vi "Track Written and Read DRAM Bytes.vi"(0 "write valid":bool, 1 "reset":bool, 5 "read valid":bool, 7 "flush":bool) -> (4 "bytes written":u64, 6 "bytes read":u64, 8 "last byte flushed":bool)   [LabVIEW 2020, in "GettingStarted_Common_148X_FPGA.lvlib"]
uses:
  GettingStarted_Common_148X_FPGA.lvlib
  <instrlib>/_niInstr/Basic Elements/v1/FPGA/Private/Count Up U64.vi
  <instrlib>/_niInstr/Basic Elements/v1/FPGA/niInstr Basic Elements v1 FPGA.lvlib
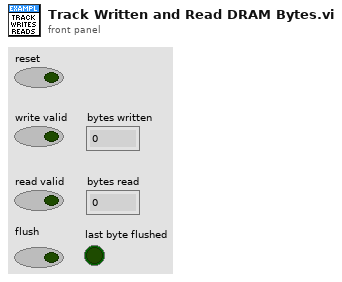
[diagram p1: front panel]
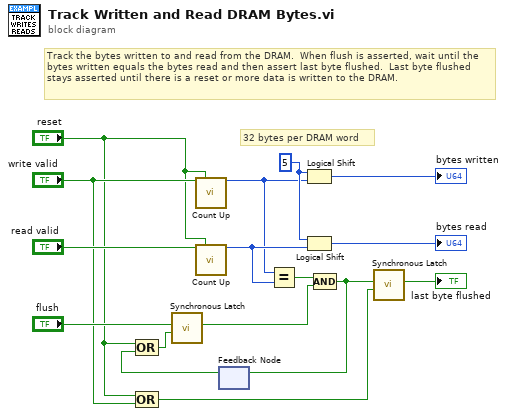
[diagram p0: block diagram]
diagram:
  w15 = i16 5 ("y")
  # "Track the bytes written to and read from the DRAM.  When flush is asserted, wait until the bytes written equals the bytes read and then assert last byte flushed.  Last byte flushed stays asserted until there is a reset or more data is written to the DRAM."
  # "32 bytes per DRAM word"
  n1 = Compound Arithmetic op=OR("reset", "write valid") -> (w7:bool)
  n2 = call-poly <instrlib>:"Count Up.vi"("increment"="write valid", "reset"="reset") -> ("count out"=w3:u64)  [unwired: 13 in]
  n3 = call-poly <instrlib>:"Count Up.vi"("increment"="read valid", "reset"="reset") -> ("count out"=w5:u64)  [unwired: 13 in]
  n4 = feedback #1() -> (w11:bool)  [unwired: 1 in]
  n5 = Compound Arithmetic op=OR("reset", w11) -> (w14:bool)
  n6 = call <instrlib>:"Synchronous Latch.vi"("clear"=w14, "set"="flush") -> ("out"=w10:bool)  [unwired: 9 in]
  n7 = Equal?(x=w3, y=w5) -> (x = y?=w12:bool)
  n8 = Logical Shift(y=w15, x=w3) -> (x << y=→"bytes written":u64)
  n9 = Logical Shift(y=w15, x=w5) -> (x << y=→"bytes read":u64)
  n10 = Compound Arithmetic op=AND(w12, w10) -> (w9:bool)
  n11 = feedback-in #1(w9) -> ()
  n12 = call <instrlib>:"Synchronous Latch.vi"("clear"=w7, "set"=w9) -> ("out"=→"last byte flushed":bool)  [unwired: 9 in]
